vi "ReadDataVariant.vi"(8 "error in (no error)":errorcluster, 11 "Singleton.lvclass In":refnum<class "Singleton.lvclass">) -> (0 "error out":errorcluster, 2 "DataVariant":variant, 3 "SingletonDVR Out":refnum<data-value>)   [LabVIEW 2014, in "Singleton.lvclass"]
uses:
  Singleton.lvclass
  Singleton.lvclass/Singleton.ctl
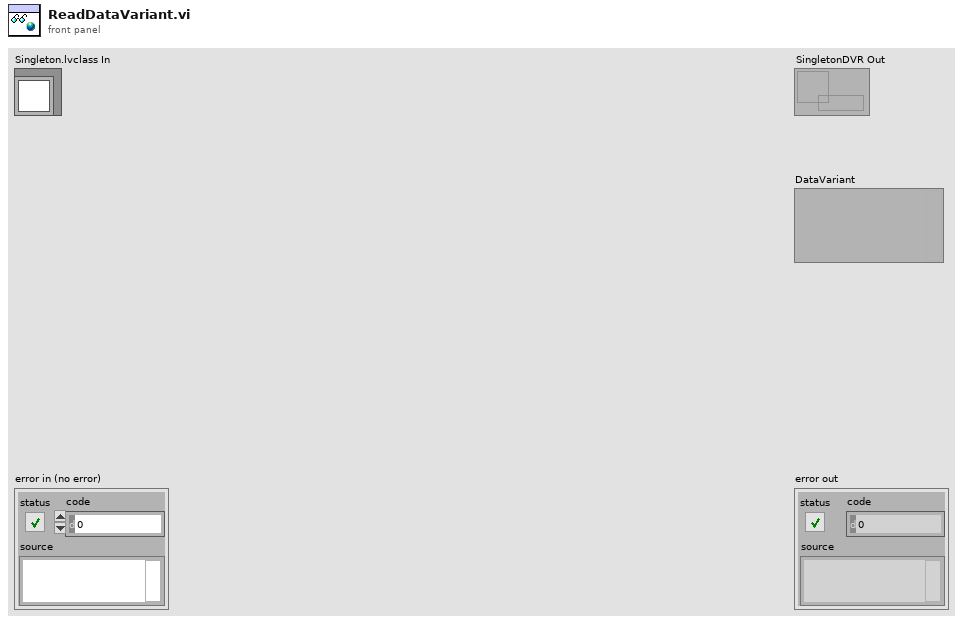
[diagram p1: front panel]
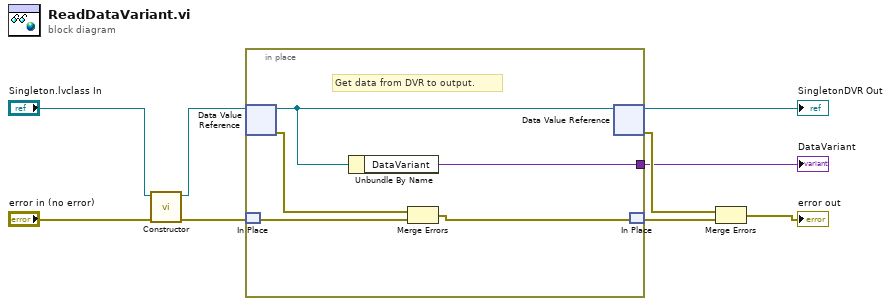
[diagram p0: block diagram]
diagram:
  n1 = call "Constructor.vi"("error in (no error)"="error in (no error)", "Singleton.lvclass In"="Singleton.lvclass In") -> ("error out"=w7:errorcluster, "SingletonDVR Out"=w8:refnum<data-value>)  [unwired: 8 in]
  n2 = in-place {
    in-place-border: [w10] -> w3
    # "Get data from DVR to output."
    n3 = in-place-dvr #1(w8) -> (w11:refnum<class "Singleton.lvclass">, w12:errorcluster)
    n4 = in-place-match #2(w7) -> (w14:errorcluster)
    n5 = Unbundle By Name(w11) -> ("DataVariant"=w10:variant)
    n6 = Merge Errors(w12, w14) -> (w13:errorcluster)
    n7 = in-place-dvr #1(w11) -> (→"SingletonDVR Out":refnum<data-value>, w5:errorcluster)
    n8 = in-place-match #2(w13) -> (w6:errorcluster)
  }
  "DataVariant" <- w3
  n9 = Merge Errors(w5, w6) -> (→"error out":errorcluster)
